vi "Hardware_Power Supplies_Analog.vi"(0 "Desired Power":dbl, 1 "Task In_1":refnum<k21>, 5 "Input Resistance":dbl, 7 "Maximum Power Limit":dbl, 11 "Error In":errorcluster, 12 "Task In_2":refnum<k21>) -> (2 "Output Voltage 1":dbl format="%0.2f", 3 "Output Current 1":dbl format="%0.2f", 4 "Task Out_1":refnum<k21>, 6 "Task Out_2":refnum<k21>, 8 "Output Power":dbl format="%#.4f", 10 "Output Resistance":dbl, 13 "Output Voltage 2":dbl format="%0.2f", 14 "Output Current 2":dbl format="%0.2f", 15 "Error Out":errorcluster)   [LabVIEW 2017]
uses:
  DAQmx Fill In Error Info.vi
  NI_AALBase.lvlib
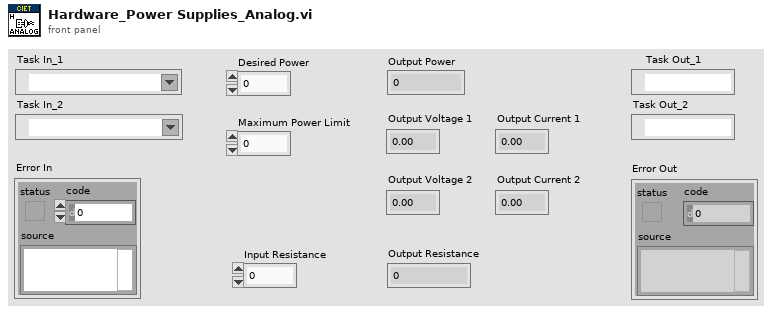
[diagram p1: front panel]
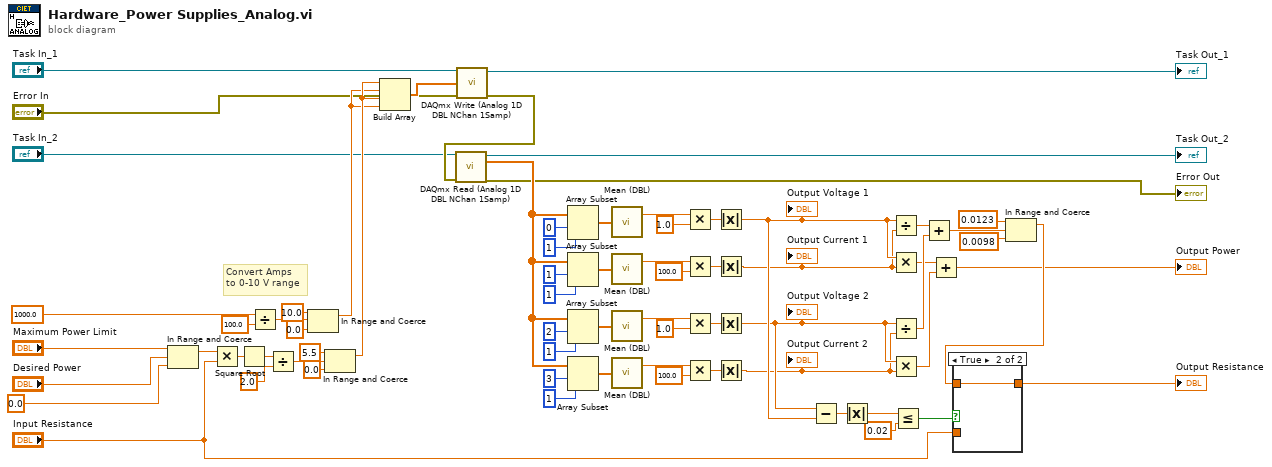
[diagram p0: block diagram]
diagram:
  # "Convert Amps \nto 0-10 V range"
  n1 = In Range and Coerce(upper limit="Maximum Power Limit", x="Desired Power", lower limit=0.0) -> (coerced(x)=w58:dbl)  [unwired: 1 out]
  n2 = Multiply(x=w58, y="Input Resistance") -> (x*y=w64:dbl)
  n3 = Square Root(x=w64) -> (sqrt(x)=w63:dbl)
  n4 = Divide(x=1000.0 ("Maximum Current Limit"), y=100.0) -> (x/y=w27:dbl)
  n5 = Divide(x=w63, y=2.0) -> (x/y=w59:dbl)
  n6 = In Range and Coerce(upper limit=10.0, x=w27, lower limit=0.0) -> (coerced(x)=w28:dbl)  [unwired: 1 out]
  n7 = In Range and Coerce(upper limit=5.5, x=w59, lower limit=0.0) -> (coerced(x)=w57:dbl)  [unwired: 1 out]
  n8 = Build Array(w57, w28, w57, w28) -> (w69:dbl[])
  n9 = call "DAQmx Write (Analog 1D DBL NChan 1Samp).vi"("task/channels in"="Task In_1", "data"=w69, "error in"="Error In") -> ("task out"=→"Task Out_1":refnum<k21>, "error out"=w68:errorcluster)  [unwired: 10 in, 1 out]
  n10 = call "DAQmx Read (Analog 1D DBL NChan 1Samp).vi"("task/channels in"="Task In_2", "error in"=w68) -> ("task out"=→"Task Out_2":refnum<k21>, "data"=w48:dbl[], "error out"=→"Error Out":errorcluster)  [unwired: 11 in]
  n11 = Array Subset(array=w48, index=0, length=1) -> (w34:dbl[])
  n12 = Array Subset(array=w48, index=1, length=1) -> (w33:dbl[])
  n13 = Array Subset(array=w48, index=2, length=1) -> (w32:dbl[])
  n14 = Array Subset(array=w48, index=3, length=1) -> (w31:dbl[])
  n15 = call "Mean (DBL).vi"("X"=w34) -> ("mean"=w22:dbl)  [unwired: 1 out]
  n16 = call "Mean (DBL).vi"("X"=w33) -> ("mean"=w18:dbl)  [unwired: 1 out]
  n17 = call "Mean (DBL).vi"("X"=w32) -> ("mean"=w20:dbl)  [unwired: 1 out]
  n18 = call "Mean (DBL).vi"("X"=w31) -> ("mean"=w16:dbl)  [unwired: 1 out]
  n19 = Multiply(x=w22, y=1.0) -> (x*y=w8:dbl)
  n20 = Multiply(x=w18, y=100.0) -> (x*y=w6:dbl)
  n21 = Multiply(x=w20, y=1.0) -> (x*y=w4:dbl)
  n22 = Multiply(x=w16, y=100.0) -> (x*y=w2:dbl)
  n23 = Absolute Value(x=w8) -> (abs(x)=w7:dbl)
  "Output Voltage 1" <- w7
  n24 = Absolute Value(x=w6) -> (abs(x)=w5:dbl)
  "Output Current 1" <- w5
  n25 = Absolute Value(x=w4) -> (abs(x)=w3:dbl)
  "Output Voltage 2" <- w3
  n26 = Absolute Value(x=w2) -> (abs(x)=w1:dbl)
  "Output Current 2" <- w1
  n27 = Subtract(x=w3, y=w7) -> (x-y=w40:dbl)
  n28 = Absolute Value(x=w40) -> (abs(x)=w42:dbl)
  n29 = Divide(x=w7, y=w5) -> (x/y=w44:dbl)
  n30 = Multiply(x=w7, y=w5) -> (x*y=w26:dbl)
  n31 = Divide(x=w3, y=w1) -> (x/y=w43:dbl)
  n32 = Multiply(x=w3, y=w1) -> (x*y=w25:dbl)
  n33 = Less Or Equal?(x=w42, y=0.02) -> (x <= y?=w39:bool)
  n34 = Add(x=w44, y=w43) -> (x+y=w45:dbl)
  n35 = Add(x=w26, y=w25) -> (x+y=→"Output Power":dbl)
  n36 = In Range and Coerce(upper limit=0.0123, x=w45, lower limit=0.0098) -> (coerced(x)=w37:dbl)  [unwired: 1 out]
  n37 = case shown="True" w39 {
    tunnel: w37 -> [_ w71]
    tunnel: [w70 w71] -> w38
    tunnel: "Input Resistance" -> [w70 _]
    frame False {
    }
    frame True {
    }
  }
  "Output Resistance" <- w38
